vi "Call VI.vi"(8 "error in (no error)":errorcluster, 9 "DVR":refnum<data-value>, 10 "Section":string, 11 "Speed Mode in":refnum<class "Speed Mode.lvclass">) -> (0 "error out":errorcluster, 1 "VI Ref":refnum<vi>, 2 "Asynch Ref":refnum<vi>, 3 "Speed Mode out":refnum<class "Speed Mode.lvclass">)   [LabVIEW 2020, in "Speed Mode.lvclass"]
uses:
  Speed Mode.lvclass
  Speed Mode.lvclass/Speed Mode.ctl
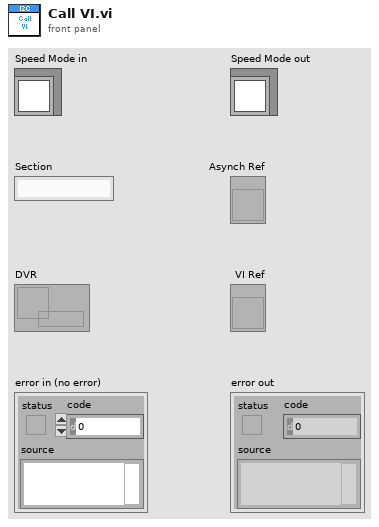
[diagram p1: front panel]
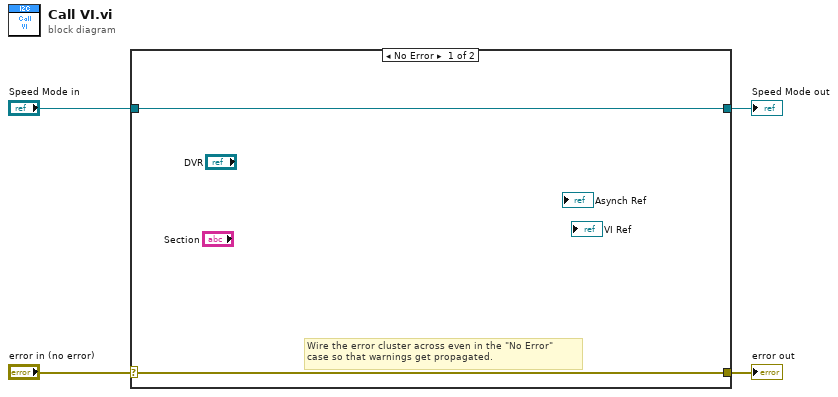
[diagram p0: block diagram]
diagram:
  n1 = case shown="No Error" "error in (no error)" {
    selector: "error in (no error)" -> [w5 w8]
    tunnel: [w5 w8] -> w3
    tunnel: [w6 w7] -> w1
    tunnel: "Speed Mode in" -> [w6 w7]
    frame No Error {
      # "Wire the error cluster across even in the \"No Error\"\ncase so that warnings get propagated."
    }
    frame Error {
    }
  }
  "error out" <- w3
  "Speed Mode out" <- w1
